vi "MQTT_Q_PVT_BuildFixedHeader.vi"(6 "Remaining Length":u32, 8 "error in (no error)":errorcluster, 11 "MessageType":T1=enum."CONNECT") -> (0 "error out":errorcluster, 3 "Fixed Header":u8[](array[numeric]))   [LabVIEW 2015, in "MQTT_Q.lvclass"]
uses:
  MQTT_Q.lvclass
  MQTT_Q_PVT_MessageType.ctl
  MQTT_Q_QoS.ctl
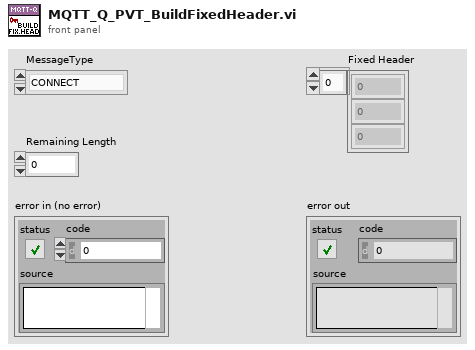
[diagram p1: front panel]
types:
  T1 = typedef "MQTT_Q.lvclass/MQTT_Q_PVT_MessageType.ctl" = enum32{"Reserved", "CONNECT", "CONNACK", "PUBLISH", "PUBACK", "PUBREC", "PUBREL", "PUBCOMP", "SUBSCRIBE", "SUBACK", "UNSUBSCRIBE", "UNSUBACK", "PINGREQ", "PINGRESP", "DISCONNECT", "Reserved2"}
  T2 = typedef "MQTT_Q.lvclass/MQTT_Q_QoS.ctl" = enum8{"At most once", "At least once", "Exactly once", "Reserved"}
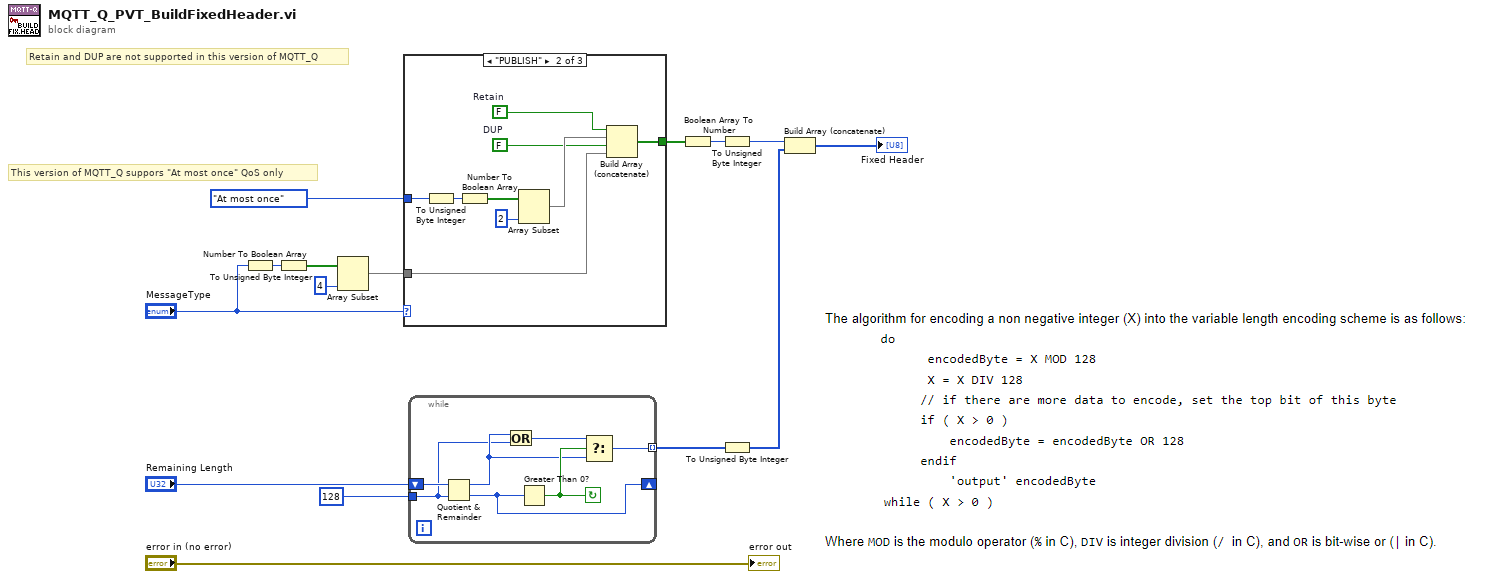
[diagram p0: block diagram]
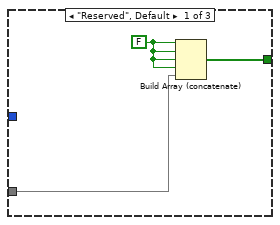
[diagram p2: hidden frame]
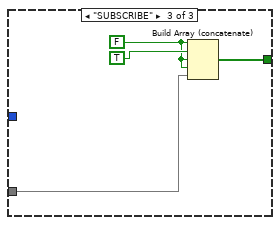
[diagram p3: hidden frame]
diagram:
  # "This version of MQTT_Q suppors \"At most once\" QoS only"
  # "Retain and DUP are not supported in this version of MQTT_Q"
  n1 = To Unsigned Byte Integer(number="MessageType") -> (unsigned 8bit integer=w15:u8)
  n2 = Number To Boolean Array(number=w15) -> (Boolean array=w14:bool[])
  n3 = Array Subset(array=w14, length=4) -> (w8:bool[])  [unwired: 1 in]
  n4 = case shown="\"PUBLISH\"" "MessageType" {
    tunnel: [w18 w27 w28] -> w6
    tunnel: MQTT_Q_QoS."At most once" ("QoS") -> [_ w22 _]
    tunnel: w8 -> [w16 w26 w31]
    frame "Reserved", Default {
      w17 = FALSE
      n5 = Build Array (concatenate)(w17, w17, w17, w17, w16) -> (w18:bool[])
    }
    frame "PUBLISH" {
      w19 = FALSE  # DUP
      w20 = FALSE  # Retain
      n6 = To Unsigned Byte Integer(number=w22) -> (unsigned 8bit integer=w23:u8)
      n7 = Number To Boolean Array(number=w23) -> (Boolean array=w24:bool[])
      n8 = Array Subset(array=w24, length=2) -> (w21:bool[])  [unwired: 1 in]
      n9 = Build Array (concatenate)(w20, w21, w19, w26) -> (w27:bool[])
    }
    frame "SUBSCRIBE" {
      w29 = FALSE
      n10 = Build Array (concatenate)(w29, TRUE, w29, w29, w31) -> (w28:bool[])
    }
  }
  n11 = while {
    shift-right: [w34] -> _
    shift-left: "Remaining Length" -> [w38]
    tunnel: [w36] -> w5 mode=indexing
    tunnel: u32 128 ("y") -> [w32]
    stop <- w37 continue-if-true
    n12 = Quotient & Remainder(x=w38, y=w32) -> (x-y*floor(x/y)=w33:u32, floor(x/y)=w34:u32)
    n13 = Or(x=w33, y=w32) -> (x .or. y?=w35:u32)
    n14 = Greater Than 0?(x=w34) -> (x > 0?=w37:bool)
    n15 = Select(t=w35, s=w37, f=w33) -> (s? t:f=w36:u32)
  }
  n16 = Boolean Array To Number(Boolean array=w6) -> (number=w12:u32)
  n17 = To Unsigned Byte Integer(number=w12) -> (unsigned 8bit integer=w11:u8)
  n18 = To Unsigned Byte Integer(number=w5) -> (unsigned 8bit integer=w3:u8[])
  n19 = Build Array (concatenate)(w11, w3) -> (→"Fixed Header":u8[])
  "error out" <- "error in (no error)"
